vi "Write.EngineData.vi"(8 "error in":errorcluster, 11 "Write in":refnum<class "Write.lvclass">) -> (0 "error out":errorcluster, 3 "Write out":refnum<class "Write.lvclass">)   [LabVIEW 2027, in "Data Access Engine (Express).lvlib" / "Write.lvclass"]
uses:
  Write.lvclass
  Write.lvclass/Write.ctl
  <userlib>/Custom Device Interfaces_v1.lvlibp/CustomDeviceAPI/Custom Device API.lvclass
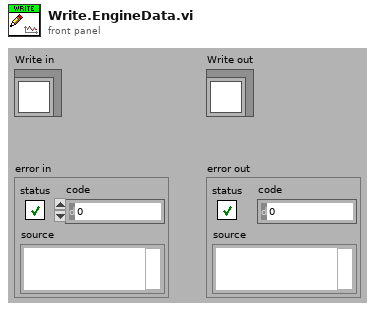
[diagram p1: front panel]
types:
  T1 = typedef "Custom Device API.lvlib/Block Data Reference.ctl" = cluster{"Data Reference":T2, "Offset":u64, "Length":u64}
  T2 = typedef "Custom Device API.lvlib/Data Reference.ctl" = i32
  T3 = cluster{"Data Reference":i32, "Offset":u64, "Length":u64}[]
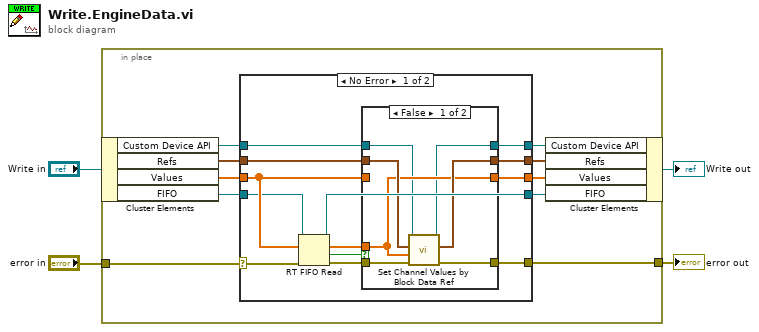
[diagram p0: block diagram]
diagram:
  n1 = in-place {
    in-place-border: [w14] -> w4
    in-place-border: "error in" -> [w9]
    n2 = in-place-cluster #1("Write in") -> ("Custom Device API"=w6:refnum<class "Custom Device API.lvclass">, "Refs"=w13:T1[], "Values"=w12:dbl[], "FIFO"=w8:refnum<k33>)
    n3 = case shown="No Error" w9 {
      selector: w9 -> [w24 w43]
      tunnel: [w27 w43] -> w14
      tunnel: [w21 w42] -> w11
      tunnel: w13 -> [w20 w41]
      tunnel: w12 -> [w22 w42]
      tunnel: [w17 w41] -> w10
      tunnel: w8 -> [w19 w40]
      tunnel: [w18 w40] -> w7
      tunnel: w6 -> [w16 w39]
      tunnel: [w15 w39] -> w5
      frame No Error {
        n4 = RT FIFO Read(0:w19, 1:w22, 3:w24) -> (8:w18:refnum<k33>, 9:w25:dbl[], 10:w23:bool, 11:w26:errorcluster)  [unwired: 1 in, 1 out]
        n5 = case shown="False" w23 {
          tunnel: w26 -> [w31 w38]
          tunnel: w25 -> [w32 _]
          tunnel: [w30 w38] -> w27
          tunnel: [w32 w37] -> w21
          tunnel: w20 -> [w34 w36]
          tunnel: w22 -> [_ w37]
          tunnel: [w33 w36] -> w17
          tunnel: w16 -> [w29 w35]
          tunnel: [w28 w35] -> w15
          frame False {
            n6 = call-dynamic "Set Channel Values by Block Data Ref.vi"("error in"=w31, "Values in"=w32, "Block Data Ref in"=w34, "Custom Device API in"=w29) -> ("error out"=w30:errorcluster, "Block Data Ref out"=w33:T3, "Custom Device API out"=w28:refnum<class "Custom Device API.lvclass">)  [unwired: 4 in, 1 out]
          }
          frame True {
          }
        }
      }
      frame Error {
      }
    }
    n7 = in-place-cluster #1("Custom Device API"=w5, "Refs"=w10, "Values"=w11, "FIFO"=w7) -> (→"Write out":refnum<class "Write.lvclass">)
  }
  "error out" <- w4
